vi "Saving Sandbox (RT).vi"() -> ()   [LabVIEW 2013]
uses:
  <vilib>/Utility/file.llb/Write To Spreadsheet File (DBL).vi
  <vilib>/NI_Real-Time Target Support.lvlib
panel:
  out "File Indicator":i32[](array[numeric])
  in  "file":i32
  out "stop":bool
  out "CPU%":dbl[](array[numeric])
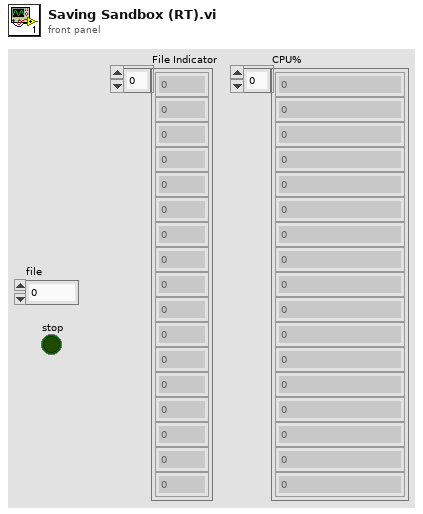
[diagram p1: front panel]
types:
  T1 = cluster{"DataNum":dbl[][], "filepath":path, "init time":dbl, "FilePaths":path[], "File#":i32, "refnum":refnum<file>}
  T2 = typedef "NI_Real-Time Target Support.lvlib/RT CPU Load.ctl" = cluster{"Total (%)":dbl, "Time Critical (%)":dbl, "Timed Structures (%)":dbl, "High (%)":dbl, "Above Normal (%)":dbl, "Normal (%)":dbl, "Background (%)":dbl, "Idle (%)":dbl, "ISR (%)":dbl}
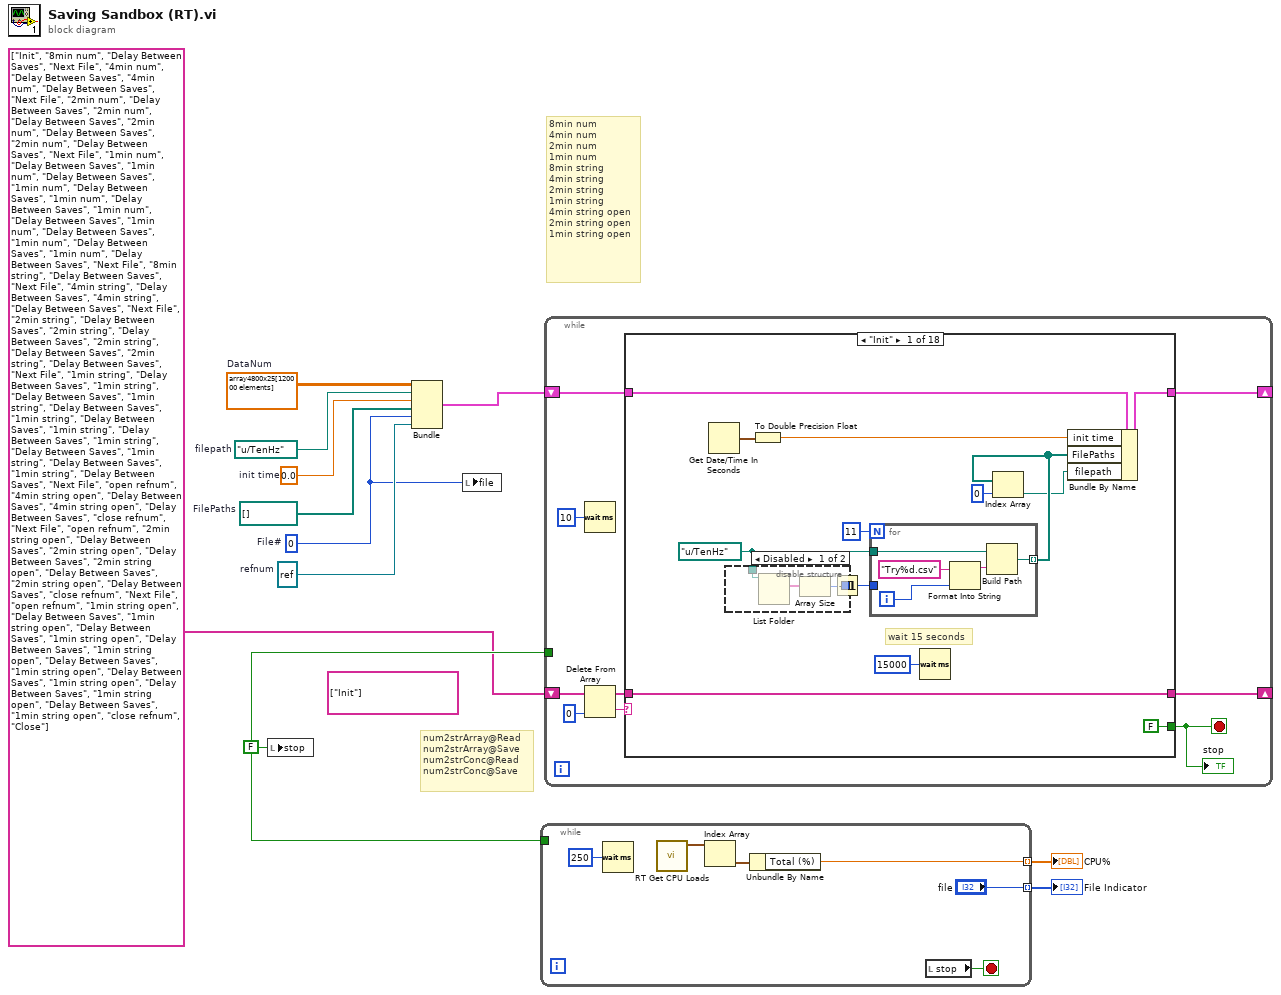
[diagram p0: block diagram]
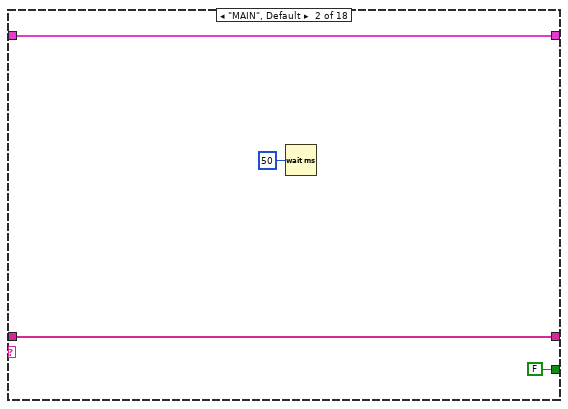
[diagram p3: hidden frame]
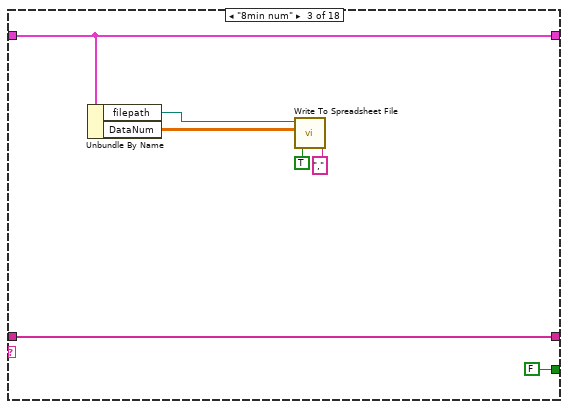
[diagram p4: hidden frame]
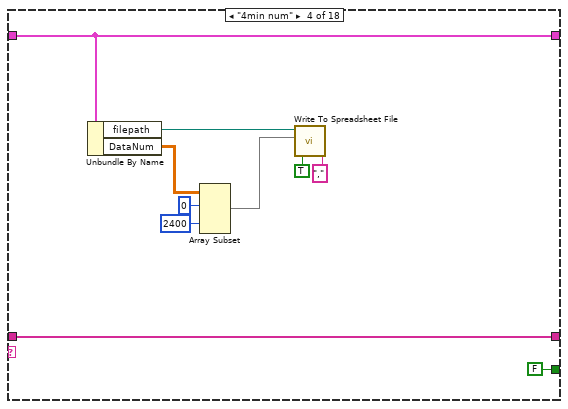
[diagram p5: hidden frame]
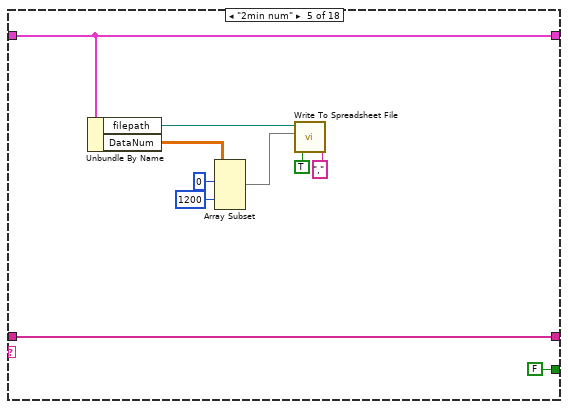
[diagram p6: hidden frame]
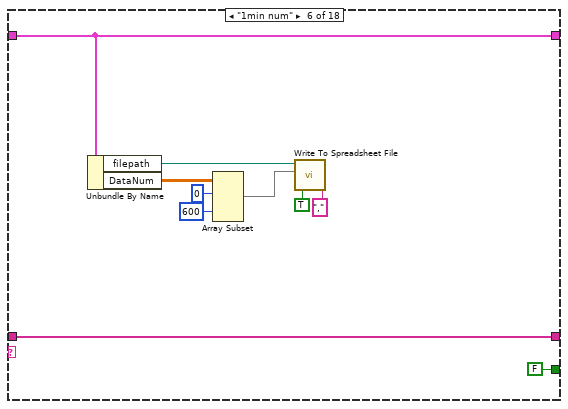
[diagram p7: hidden frame]
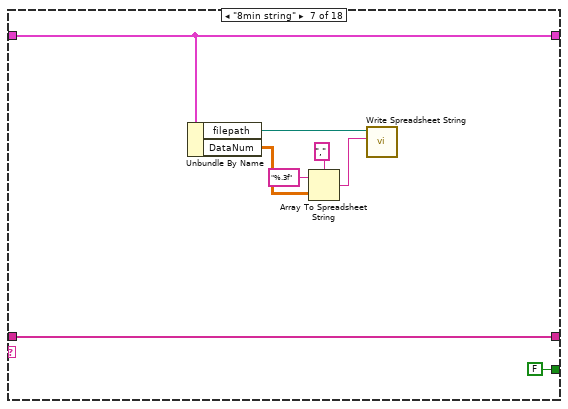
[diagram p8: hidden frame]
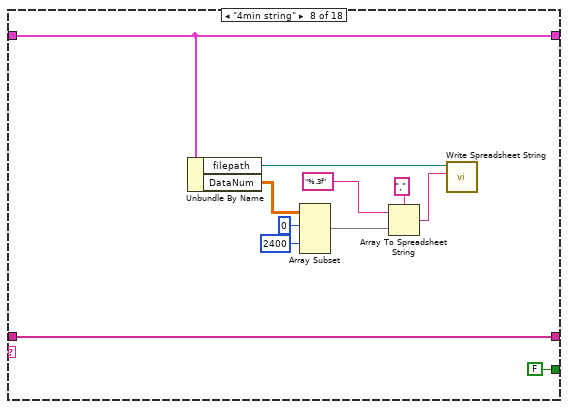
[diagram p9: hidden frame]
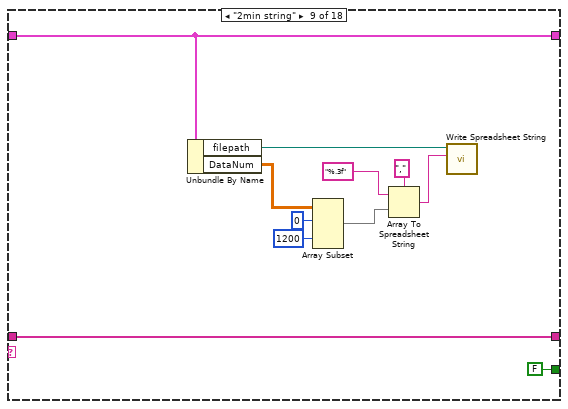
[diagram p10: hidden frame]
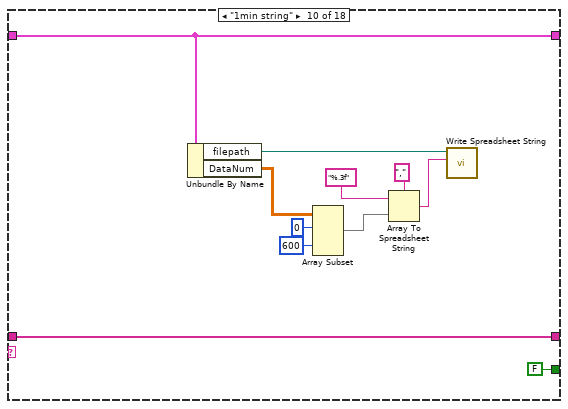
[diagram p11: hidden frame]
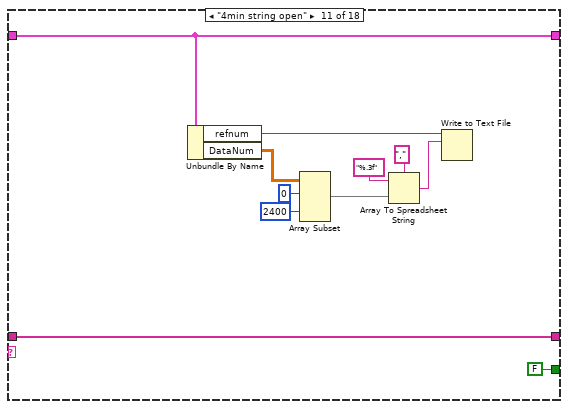
[diagram p12: hidden frame]
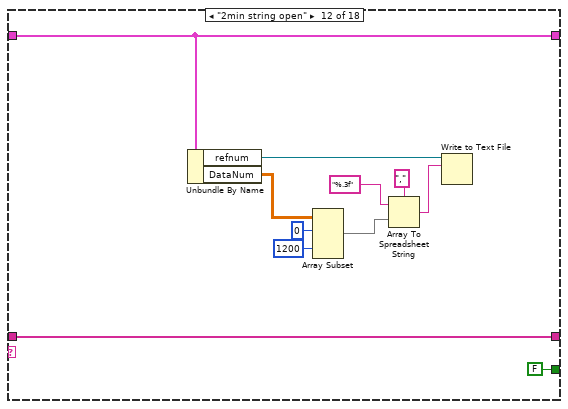
[diagram p13: hidden frame]
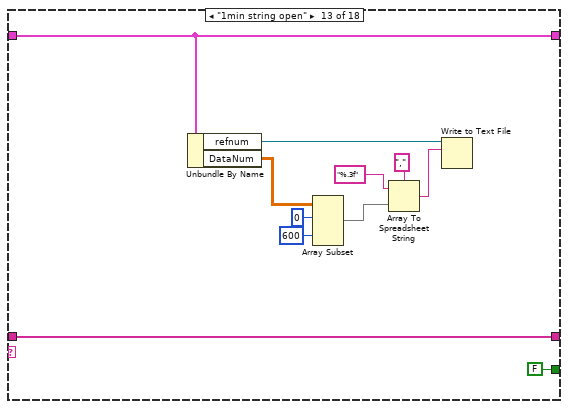
[diagram p14: hidden frame]
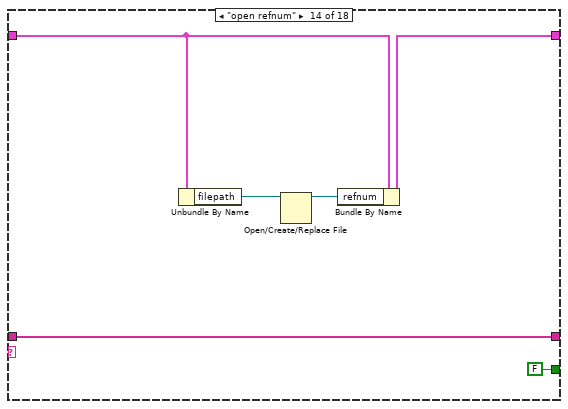
[diagram p15: hidden frame]
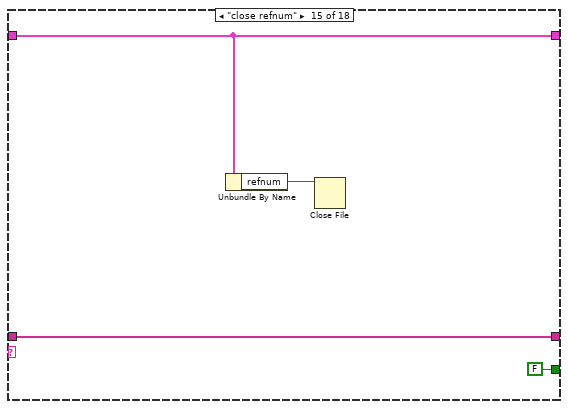
[diagram p16: hidden frame]
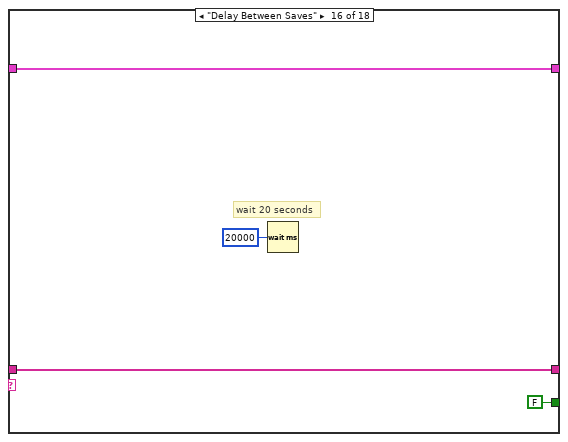
[diagram p17: hidden frame]
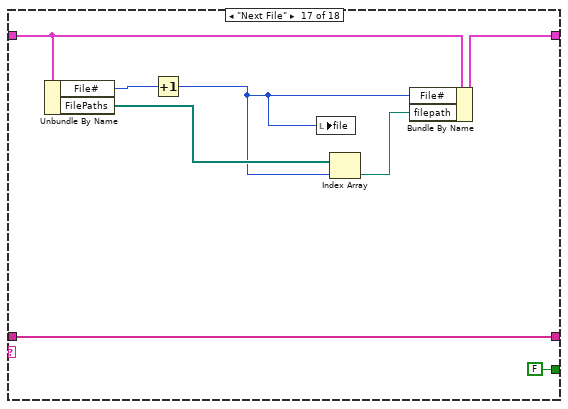
[diagram p18: hidden frame]
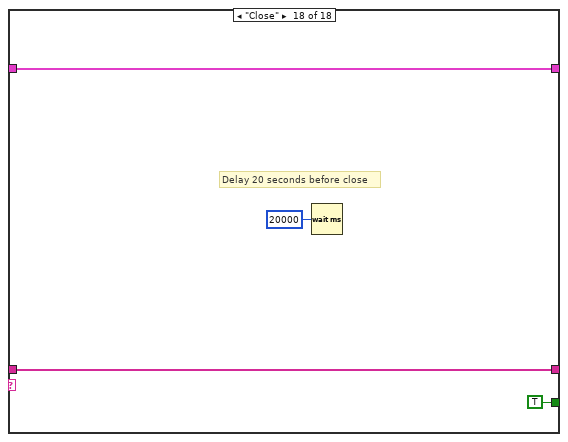
[diagram p19: hidden frame]
diagram:
  w4 = refnum<file> refnum  # refnum
  w2 = 0  # File#
  w5 = path[] []  # FilePaths
  w6 = dbl[][] array4800x25[120000 elements]  # DataNum
  w7 = 0.0  # init time
  w8 = FALSE ("stop")
  w10 = path "u:/TenHz"  # filepath
  (unwired) string[] ["Init"]
  # "8min num\n4min num\n2min num\n1min num\n8min string\n4min string\n2min string\n1min string\n4min string open\n2min string open\n1min string open"
  # "num2strArray@Read\nnum2strArray@Save\nnum2strConc@Read\nnum2strConc@Save"
  n1 = local write "stop"(w8) -> ()
  n2 = Bundle("DataNum"=w6, "filepath"=w10, "init time"=w7, "FilePaths"=w5, "File#"=w2, "refnum"=w4) -> (w11:T1)  [unwired: 1 in]
  n3 = local write "file"(w2) -> ()
  n4 = while {
    tunnel: [w13] -> w9 mode=indexing
    tunnel: w8 -> [_]
    tunnel: ["file"] -> w1 mode=indexing
    stop <- w14 stop-if-true
    n5 = Wait (ms)(milliseconds to wait=u32 250) -> ()  [unwired: 1 out]
    n6 = call <vilib>:"RT Get CPU Loads.vi"() -> ("CPU loads"=w17:T2[])  [unwired: 10 in, 1 out]
    n7 = Index Array(array=w17) -> (element=w16:T2)  [unwired: 1 in]
    n8 = Unbundle By Name(w16) -> ("Total (%)"=w13:dbl)
    n9 = local read "stop"() -> (w14:bool)
  }
  "CPU%" <- w9
  "File Indicator" <- w1
  n10 = while {
    shift-right: [w22] -> _
    shift-left: string[] ["Init", "8min num", "Delay Between Saves", "Next File", "4min num", "Delay Between Saves", "4min num", "Delay Between Saves", "Next File", "2min num", "Delay Between Saves", "2min num", "Delay Between Saves", "2min num", "Delay Between Saves", "2min num", "Delay Between Saves", "Next File", "1min num", "Delay Between Saves", "1min num", "Delay Between Saves", "1min num", "Delay Between Saves", "1min num", "Delay Between Saves", "1min num", "Delay Between Saves", "1min num", "Delay Between Saves", "1min num", "Delay Between Saves", "1min num", "Delay Between Saves", "Next File", "8min string", "Delay Between Saves", "Next File", "4min string", "Delay Between Saves", "4min string", "Delay Between Saves", "Next File", "2min string", "Delay Between Saves", "2min string", "Delay Between Saves", "2min string", "Delay Between Saves", "2min string", "Delay Between Saves", "Next File", "1min string", "Delay Between Saves", "1min string", "Delay Between Saves", "1min string", "Delay Between Saves", "1min string", "Delay Between Saves", "1min string", "Delay Between Saves", "1min string", "Delay Between Saves", "1min string", "Delay Between Saves", "1min string", "Delay Between Saves", "Next File", "open refnum", "4min string open", "Delay Between Saves", "4min string open", "Delay Between Saves", "close refnum", "Next File", "open refnum", "2min string open", "Delay Between Saves", "2min string open", "Delay Between Saves", "2min string open", "Delay Between Saves", "2min string open", "Delay Between Saves", "close refnum", "Next File", "open refnum", "1min string open", "Delay Between Saves", "1min string open", "Delay Between Saves", "1min string open", "Delay Between Saves", "1min string open", "Delay Between Saves", "1min string open", "Delay Between Saves", "1min string open", "Delay Between Saves", "1min string open", "Delay Between Saves", "1min string open", "close refnum", "Close"] -> [w26]
    shift-right: [w20] -> _
    shift-left: w11 -> [w21]
    tunnel: w8 -> [_]
    stop <- w18 stop-if-true
    n11 = Wait (ms)(milliseconds to wait=u32 10) -> ()  [unwired: 1 out]
    n12 = Delete From Array(array=w26, index=0) -> (deleted portion=w24:string, array with subset deleted=w23:string[])  [unwired: 1 in]
    n13 = case shown="\"Init\"" w24 {
      tunnel: [w36 w50 w53 w66 w75 w81 w95 w100 w111 w122 w135 w146 w157 w169 w173 w176 w185 w188] -> w22
      tunnel: w23 -> [w36 w50 w53 w66 w75 w81 w95 w100 w111 w122 w135 w146 w157 w169 w173 w176 w185 w188]
      tunnel: [w37 w51 w57 w65 w76 w82 w96 w101 w112 w123 w136 w147 w158 w165 w172 w177 w182 w187] -> w20
      tunnel: w21 -> [w38 w51 w57 w65 w76 w82 w96 w101 w112 w123 w136 w147 w158 w166 w172 w177 w183 w187]
      tunnel: [FALSE FALSE FALSE FALSE FALSE FALSE FALSE FALSE FALSE FALSE FALSE FALSE FALSE FALSE FALSE FALSE FALSE TRUE] -> w18
      frame "Init" {
        w34 = path "u:/TenHz"
        # "wait 15 seconds"
        n14 = Get Date/Time In Seconds() -> (seconds since 1Jan1904=w39:timestamp)
        n15 = disable-structure shown="Disabled" {
          disable-tunnel: [w48 _] -> w35
          disable-tunnel: w34 -> [w47 _]
          frame Disabled {
            n16 = List Folder(path=w47) -> (filenames=w45:string[])  [unwired: 3 in, 3 out]
            n17 = Array Size(array=w45) -> (size(s)=w46:i32)
            n18 = Increment(x=w46) -> (x+1=w48:i32)
          }
          frame Enabled {
          }
        }
        n19 = To Double Precision Float(number=w39) -> (double precision float=w32:dbl)
        n20 = for {
          N: 11 -> [_]
          tunnel: w35 -> [_]
          tunnel: w34 -> [w42]
          tunnel: [w41] -> w29 mode=indexing
          i -> [w40]
          n21 = Format Into String(format string="Try%d.csv" ("initial string"), w40) -> (resulting string=w43:string)  [unwired: 2 in, 1 out]
          n22 = Build Path(base path=w42, name or relative path=w43) -> (appended path=w41:path)
        }
        n23 = Wait (ms)(milliseconds to wait=u32 15000) -> ()  [unwired: 1 out]
        n24 = Index Array(array=w29, index=0) -> (element=w27:path)
        n25 = Bundle By Name(cluster=w38, "init time"=w32, "FilePaths"=w29, "filepath"=w27) -> (w37:T1)
      }
      frame "MAIN", Default {
        n26 = Wait (ms)(milliseconds to wait=u32 50) -> ()  [unwired: 1 out]
      }
      frame "8min num" {
        n27 = Unbundle By Name(w57) -> ("filepath"=w56:path, "DataNum"=w55:dbl[][])
        n28 = call-poly <vilib>:"Write To Spreadsheet File.vi"("delimiter (\\t)"="," ("delimiter (\\t)"), "append to file? (new file:F)"=TRUE, "2D data"=w55, "file path (dialog if empty)"=w56) -> ()  [unwired: 4 in, 1 out]
      }
      frame "4min num" {
        n29 = Unbundle By Name(w65) -> ("filepath"=w67:path, "DataNum"=w64:dbl[][])
        n30 = Array Subset(array=w64, index (row)=0 ("index"), length (row)=2400 ("length")) -> (w61:dbl[][])  [unwired: 2 in]
        n31 = call-poly <vilib>:"Write To Spreadsheet File.vi"("delimiter (\\t)"="," ("delimiter (\\t)"), "append to file? (new file:F)"=TRUE, "2D data"=w61, "file path (dialog if empty)"=w67) -> ()  [unwired: 4 in, 1 out]
      }
      frame "2min num" {
        n32 = Unbundle By Name(w76) -> ("filepath"=w77:path, "DataNum"=w72:dbl[][])
        n33 = Array Subset(array=w72, index (row)=0 ("index"), length (row)=1200 ("length")) -> (w71:dbl[][])  [unwired: 2 in]
        n34 = call-poly <vilib>:"Write To Spreadsheet File.vi"("delimiter (\\t)"="," ("delimiter (\\t)"), "append to file? (new file:F)"=TRUE, "2D data"=w71, "file path (dialog if empty)"=w77) -> ()  [unwired: 4 in, 1 out]
      }
      frame "1min num" {
        n35 = Unbundle By Name(w82) -> ("filepath"=w87:path, "DataNum"=w84:dbl[][])
        n36 = Array Subset(array=w84, index (row)=0 ("index"), length (row)=600 ("length")) -> (w83:dbl[][])  [unwired: 2 in]
        n37 = call-poly <vilib>:"Write To Spreadsheet File.vi"("delimiter (\\t)"="," ("delimiter (\\t)"), "append to file? (new file:F)"=TRUE, "2D data"=w83, "file path (dialog if empty)"=w87) -> ()  [unwired: 4 in, 1 out]
      }
      frame "8min string" {
        n38 = Unbundle By Name(w96) -> ("filepath"=w91:path, "DataNum"=w94:dbl[][])
        n39 = Array To Spreadsheet String(delimiter (Tab)=",", array=w94, 3:"%.3f" ("format string")) -> (spreadsheet string=w92:string)
        n40 = call <vilib>:"Write Spreadsheet String.vi"("spreadsheet string"=w92, "file path (dialog if empty)"=w91) -> ()  [unwired: 8 in, 2 out]
      }
      frame "4min string" {
        n41 = Unbundle By Name(w101) -> ("filepath"=w106:path, "DataNum"=w103:dbl[][])
        n42 = Array Subset(array=w103, index (row)=0 ("index"), length (row)=2400 ("length")) -> (w102:dbl[][])  [unwired: 2 in]
        n43 = Array To Spreadsheet String(delimiter (Tab)=",", array=w102, 3:"%.3f" ("format string")) -> (spreadsheet string=w107:string)
        n44 = call <vilib>:"Write Spreadsheet String.vi"("spreadsheet string"=w107, "file path (dialog if empty)"=w106) -> ()  [unwired: 8 in, 2 out]
      }
      frame "2min string" {
        n45 = Unbundle By Name(w112) -> ("filepath"=w117:path, "DataNum"=w114:dbl[][])
        n46 = Array Subset(array=w114, index (row)=0 ("index"), length (row)=1200 ("length")) -> (w113:dbl[][])  [unwired: 2 in]
        n47 = Array To Spreadsheet String(delimiter (Tab)=",", array=w113, 3:"%.3f" ("format string")) -> (spreadsheet string=w118:string)
        n48 = call <vilib>:"Write Spreadsheet String.vi"("spreadsheet string"=w118, "file path (dialog if empty)"=w117) -> ()  [unwired: 8 in, 2 out]
      }
      frame "1min string" {
        n49 = Unbundle By Name(w123) -> ("filepath"=w128:path, "DataNum"=w125:dbl[][])
        n50 = Array Subset(array=w125, index (row)=0 ("index"), length (row)=600 ("length")) -> (w124:dbl[][])  [unwired: 2 in]
        n51 = Array To Spreadsheet String(delimiter (Tab)=",", array=w124, 3:"%.3f" ("format string")) -> (spreadsheet string=w129:string)
        n52 = call <vilib>:"Write Spreadsheet String.vi"("spreadsheet string"=w129, "file path (dialog if empty)"=w128) -> ()  [unwired: 8 in, 2 out]
      }
      frame "4min string open" {
        n53 = Unbundle By Name(w136) -> ("refnum"=w133:refnum<file>, "DataNum"=w138:dbl[][])
        n54 = Array Subset(array=w138, index (row)=0 ("index"), length (row)=2400 ("length")) -> (w137:dbl[][])  [unwired: 2 in]
        n55 = Array To Spreadsheet String(delimiter (Tab)=",", array=w137, 3:"%.3f" ("format string")) -> (spreadsheet string=w132:string)
        n56 = Write to Text File(file (use dialog)=w133, text=w132) -> ()  [unwired: 2 in, 3 out]
      }
      frame "2min string open" {
        n57 = Unbundle By Name(w147) -> ("refnum"=w144:refnum<file>, "DataNum"=w149:dbl[][])
        n58 = Array Subset(array=w149, index (row)=0 ("index"), length (row)=1200 ("length")) -> (w148:dbl[][])  [unwired: 2 in]
        n59 = Array To Spreadsheet String(delimiter (Tab)=",", array=w148, 3:"%.3f" ("format string")) -> (spreadsheet string=w143:string)
        n60 = Write to Text File(file (use dialog)=w144, text=w143) -> ()  [unwired: 2 in, 3 out]
      }
      frame "1min string open" {
        n61 = Unbundle By Name(w158) -> ("refnum"=w154:refnum<file>, "DataNum"=w160:dbl[][])
        n62 = Array Subset(array=w160, index (row)=0 ("index"), length (row)=600 ("length")) -> (w159:dbl[][])  [unwired: 2 in]
        n63 = Array To Spreadsheet String(delimiter (Tab)=",", array=w159, 3:"%.3f" ("format string")) -> (spreadsheet string=w155:string)
        n64 = Write to Text File(file (use dialog)=w154, text=w155) -> ()  [unwired: 2 in, 3 out]
      }
      frame "open refnum" {
        n65 = Unbundle By Name(w166) -> ("filepath"=w168:path)
        n66 = Open/Create/Replace File(file path (use dialog)=w168) -> (refnum out=w167:refnum<file>)  [unwired: 5 in, 2 out]
        n67 = Bundle By Name(cluster=w166, "refnum"=w167) -> (w165:T1)
      }
      frame "close refnum" {
        n68 = Unbundle By Name(w172) -> ("refnum"=w171:refnum<file>)
        n69 = Close File(refnum=w171) -> ()  [unwired: 1 in, 2 out]
      }
      frame "Delay Between Saves" {
        # "wait 20 seconds"
        n70 = Wait (ms)(milliseconds to wait=u32 20000) -> ()  [unwired: 1 out]
      }
      frame "Next File" {
        n71 = Unbundle By Name(w183) -> ("File#"=w181:i32, "FilePaths"=w180:path[])
        n72 = Increment(x=w181) -> (x+1=w178:i32)
        n73 = local write "file"(w178) -> ()
        n74 = Index Array(array=w180, index=w178) -> (element=w179:path)
        n75 = Bundle By Name(cluster=w183, "File#"=w178, "filepath"=w179) -> (w182:T1)
      }
      frame "Close" {
        # "Delay 20 seconds before close"
        n76 = Wait (ms)(milliseconds to wait=u32 20000) -> ()  [unwired: 1 out]
      }
    }
    "stop" <- w18
  }
